vi "Solve Linear Equations (U64).vi"(10 "b":u64[](array[numeric]), 11 "A":u64[][](array[numeric])) -> (2 "Out of Tolerance?":bool, 3 "X":u64[](array[numeric]))   [LabVIEW 2025, in "AOC.lvlib"]
uses:
  AOC.lvlib
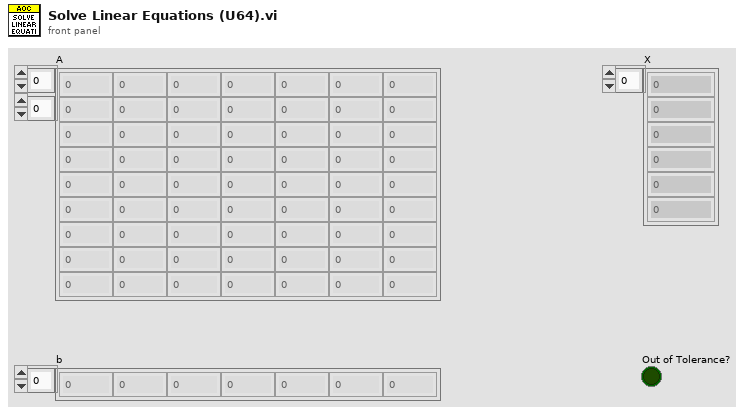
[diagram p1: front panel]
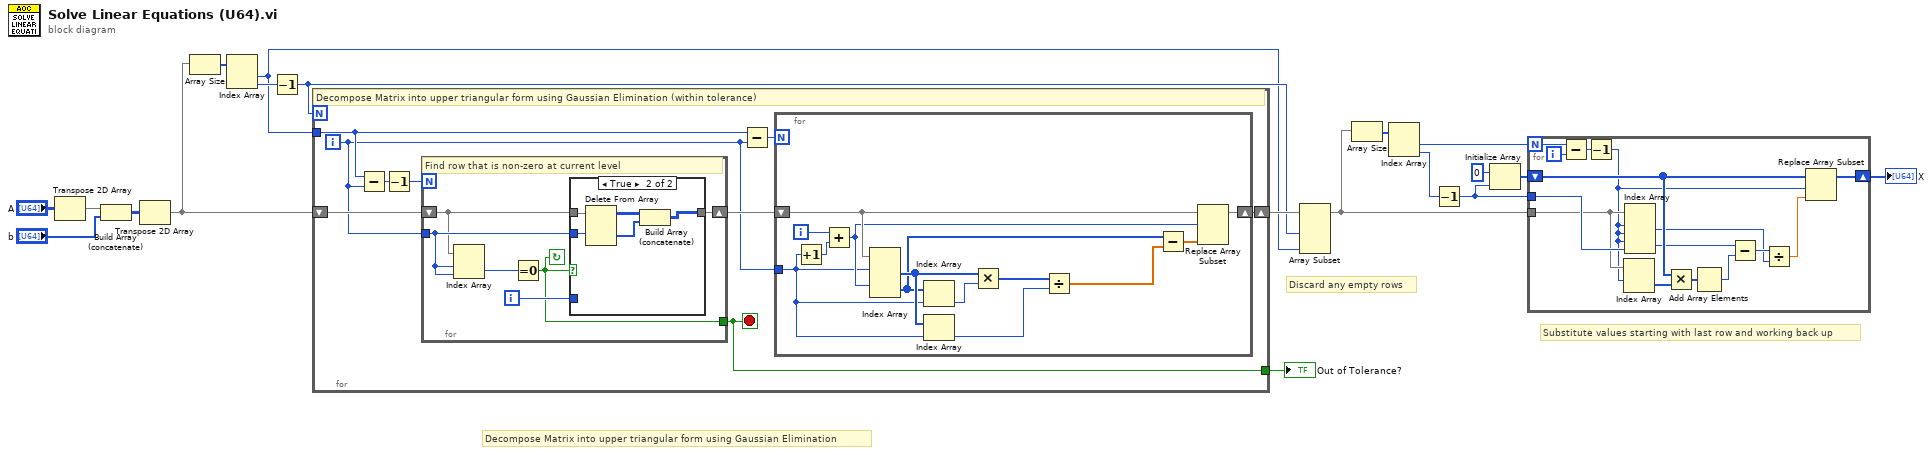
[diagram p0: block diagram]
diagram:
  # "Discard any empty rows"
  # "Substitute values starting with last row and working back up"
  # "Decompose Matrix into upper triangular form using Gaussian Elimination"
  n1 = Transpose 2D Array(2D array="A") -> (transposed array=w4:u64[][])
  n2 = Build Array (concatenate)(w4, "b") -> (w3:u64[][])
  n3 = Transpose 2D Array(2D array=w3) -> (transposed array=w2:u64[][])
  n4 = Array Size(array=w2) -> (size(s)=w19:i32[])
  n5 = Index Array(array=w19) -> (element #1=w8:i32, element #2=w18:i32)  [unwired: 2 in]
  n6 = Decrement(x=w18) -> (x-1=w9:i32)
  n7 = for {
    N: w9 -> [_]
    tunnel: w8 -> [w24]
    shift-right: [w28] -> w17
    shift-left: w2 -> [w26]
    tunnel: [w20] -> w1
    i -> [w23]
    stop <- w20 stop-if-true
    # "Decompose Matrix into upper triangular form using Gaussian Elimination (within tolerance)"
    n8 = Subtract(x=w24, y=w23) -> (x-y=w22:i32)
    n9 = Decrement(x=w22) -> (x-1=w21:i32)
    n10 = for {
      N: w21 -> [_]
      tunnel: w23 -> [w34]
      shift-right: [w32] -> w25
      shift-left: w26 -> [w33]
      tunnel: [w30] -> w20
      i -> [w31]
      stop <- w30 continue-if-true
      # "Find row that is non-zero at current level"
      n11 = Index Array(array=w33, index (row)=w34, index (col)=w34) -> (element=w29:u64)
      n12 = Equal To 0?(x=w29) -> (x = 0?=w30:bool)
      n13 = case shown="True" w30 {
        tunnel: w34 -> [_ w39]
        tunnel: w33 -> [w35 w40]
        tunnel: [w35 w36] -> w32
        tunnel: w31 -> [_ _]
        frame False {
        }
        frame True {
          n14 = Delete From Array(array=w40, index (row)=w39) -> (deleted portion=w37:u64[], array with subset deleted=w38:u64[][])  [unwired: 2 in]
          n15 = Build Array (concatenate)(w38, w37) -> (w36:u64[][])
        }
      }
    }
    n16 = Subtract(x=w24, y=w23) -> (x-y=w27:i32)
    n17 = for {
      N: w27 -> [_]
      tunnel: w23 -> [w45]
      shift-right: [w50] -> w28
      shift-left: w25 -> [w51]
      i -> [w47]
      n18 = Increment(x=w45) -> (x+1=w46:i32)
      n19 = Add(x=w47, y=w46) -> (x+y=w48:i32)
      n20 = Index Array(array=w51, index (row) #1=w45, index (row) #2=w48) -> (element #1=w53:u64[], element #2=w52:u64[])  [unwired: 2 in]
      n21 = Index Array(array=w52, index=w45) -> (element=w44:u64)
      n22 = Index Array(array=w53, index=w45) -> (element=w41:u64)
      n23 = Multiply(x=w53, y=w44) -> (x*y=w42:u64[])
      n24 = Divide(x=w42, y=w41) -> (x/y=w43:dbl[])
      n25 = Subtract(x=w52, y=w43) -> (x-y=w49:dbl[])
      n26 = Replace Array Subset(array=w51, new element=w49, index (row)=w48) -> (w50:u64[][])  [unwired: 1 in]
    }
  }
  "Out of Tolerance?" <- w1
  n27 = Array Subset(array=w17, length (row)=w9, length (col)=w8) -> (w10:u64[][])  [unwired: 2 in]
  n28 = Array Size(array=w10) -> (size(s)=w16:i32[])
  n29 = Index Array(array=w16) -> (element #1=w15:i32, element #2=w7:i32)  [unwired: 2 in]
  n30 = Decrement(x=w7) -> (x-1=w6:i32)
  n31 = Initialize Array(u64 0, w6) -> (w12:u64[])
  n32 = for {
    N: w15 -> [w68]
    tunnel: w10 -> [w62]
    tunnel: w6 -> [w66]
    shift-right: [w65] -> w14
    shift-left: w12 -> [w64]
    i -> [w67]
    n33 = Subtract(x=w68, y=w67) -> (x-y=w59:i32)
    n34 = Decrement(x=w59) -> (x-1=w58:i32)
    n35 = Index Array(array=w62, index (row)=w58) -> (element=w61:u64[])  [unwired: 1 in]
    n36 = Index Array(array=w62, index (row) #1=w58, index (col) #1=w58, index (row) #2=w58, index (col) #2=w66) -> (element #1=w54:u64, element #2=w56:u64)
    n37 = Multiply(x=w64, y=w61) -> (x*y=w63:u64[])
    n38 = Add Array Elements(numeric array=w63) -> (sum=w55:u64)
    n39 = Subtract(x=w56, y=w55) -> (x-y=w57:u64)
    n40 = Divide(x=w57, y=w54) -> (x/y=w60:dbl)
    n41 = Replace Array Subset(array=w64, new element=w60, index=w58) -> (w65:u64[])
  }
  "X" <- w14
